vi "smartmeshIP serial mux IO.vi"(5 "tx_commandType":u8(ring) items=["subscribe"=22, "startNetwork"=45, "setUser"=58, "setTime"=54, "setNetworkConfig"=26, "setLicense"=56, "setIPConfig"=68, "setDownstreamFrameMode"=51, "setCommonJoinKey"=66, "setAdvertising"=50, "setACLEntry"=39, "sendIP"=59, "sendData"=44, "restorFactoryDefaults"=61, "reset"=21, "radiotestTx"=35, "radiotestRx"=37, "pingMote"=42, "getTime"=23, "getSystemInfo"=46, "radiotestStatistics"=38, "getPathInfo"=48, "getNextPath"=49, "getNextACLEntry"=40, "getNetworkInfo"=64, "getNetworkConfig"=63, "getMoteLinks"=70, "getMoteInfo"=62, "getMoteConfigByld"=65, "getMoteConfig"=47, "getManagerStatistics"=53, "getLog"=43, "getLicense"=55, "getIPConfig"=67, "exchangeNetworkID"=34, "exchangeMoteJoinKey"=33, "deleteMote"=69, "deleteACLEntry"=41, "clearStatistics"=31], 7 "State":u16(ring) items=["Connect", "Write", "Read", "Close"], 8 "error in":errorcluster, 9 "MAC source":string="\u0000\u0017\r\u0000\u0000`#Ò", 10 "tx_data":string, 11 "serial mux adress":T1={"serial_mux IP"="127.0.0.1", "rserial_mux port"=9900}) -> (0 "error out":errorcluster, 1 "tx packet":string, 2 "rx_commandType":u8, 3 "rx_data":string, 4 "all inputs":string[](array[string]), 6 "sec since last packet":dbl)   [LabVIEW 2017]
panel:
  in  "reset connection each month?":bool=TRUE
  out "Array 2":u8[](array[numeric])
  in  "MAC destination":string="\u0000\u0017\r\u0000\u0000`#Ò"
  in  "Path ID":u16
  in  "advertising":bool
  in  "next mote on list?":bool
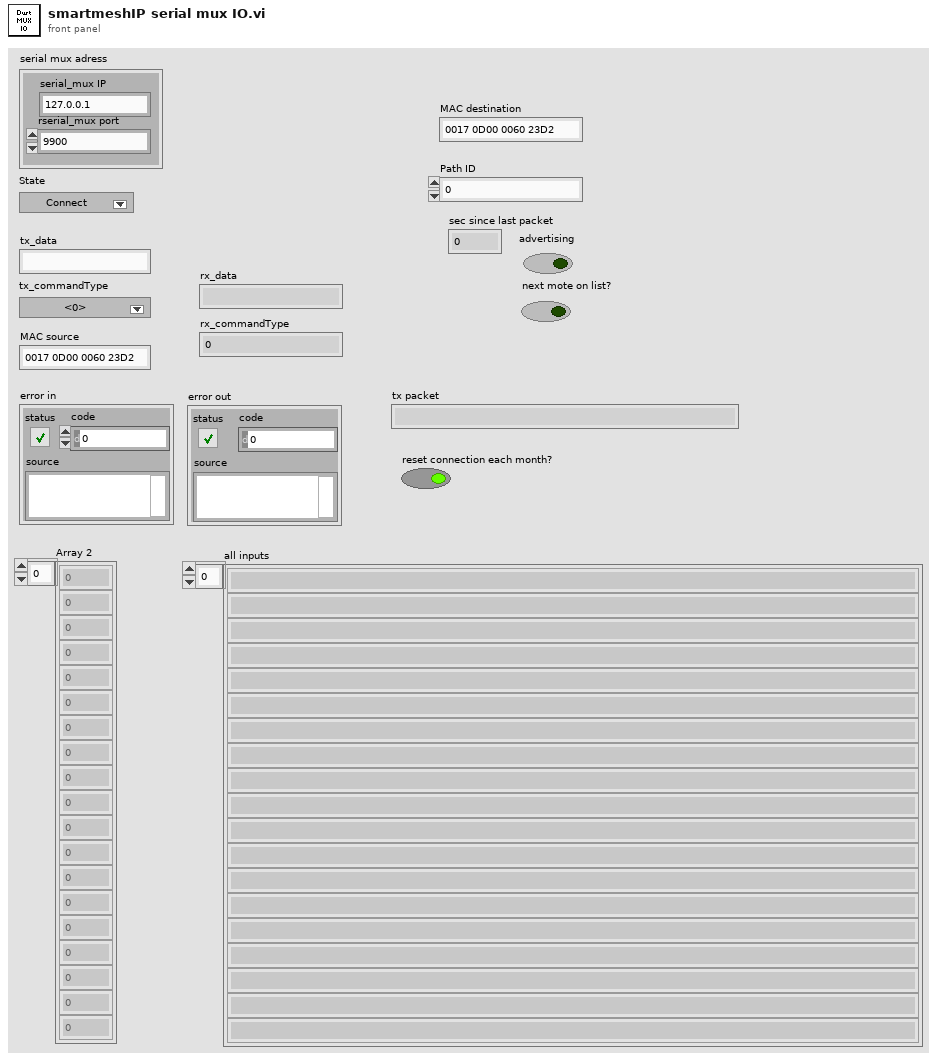
[diagram p1: front panel]
types:
  T1 = cluster{"serial_mux IP":string, "rserial_mux port":u16}
  T2 = enum16{"Standard", "Buffered", "CRLF", "Immediate"}
  T3 = typedef "LVDateTimeRec.ctl" = cluster{"fractional second":dbl, "second":i32, "minute":i32, "hour":i32, "day of month":i32, "month":i32, "year":i32, "day of week":i32, "day of year":i32, "DST":i32}
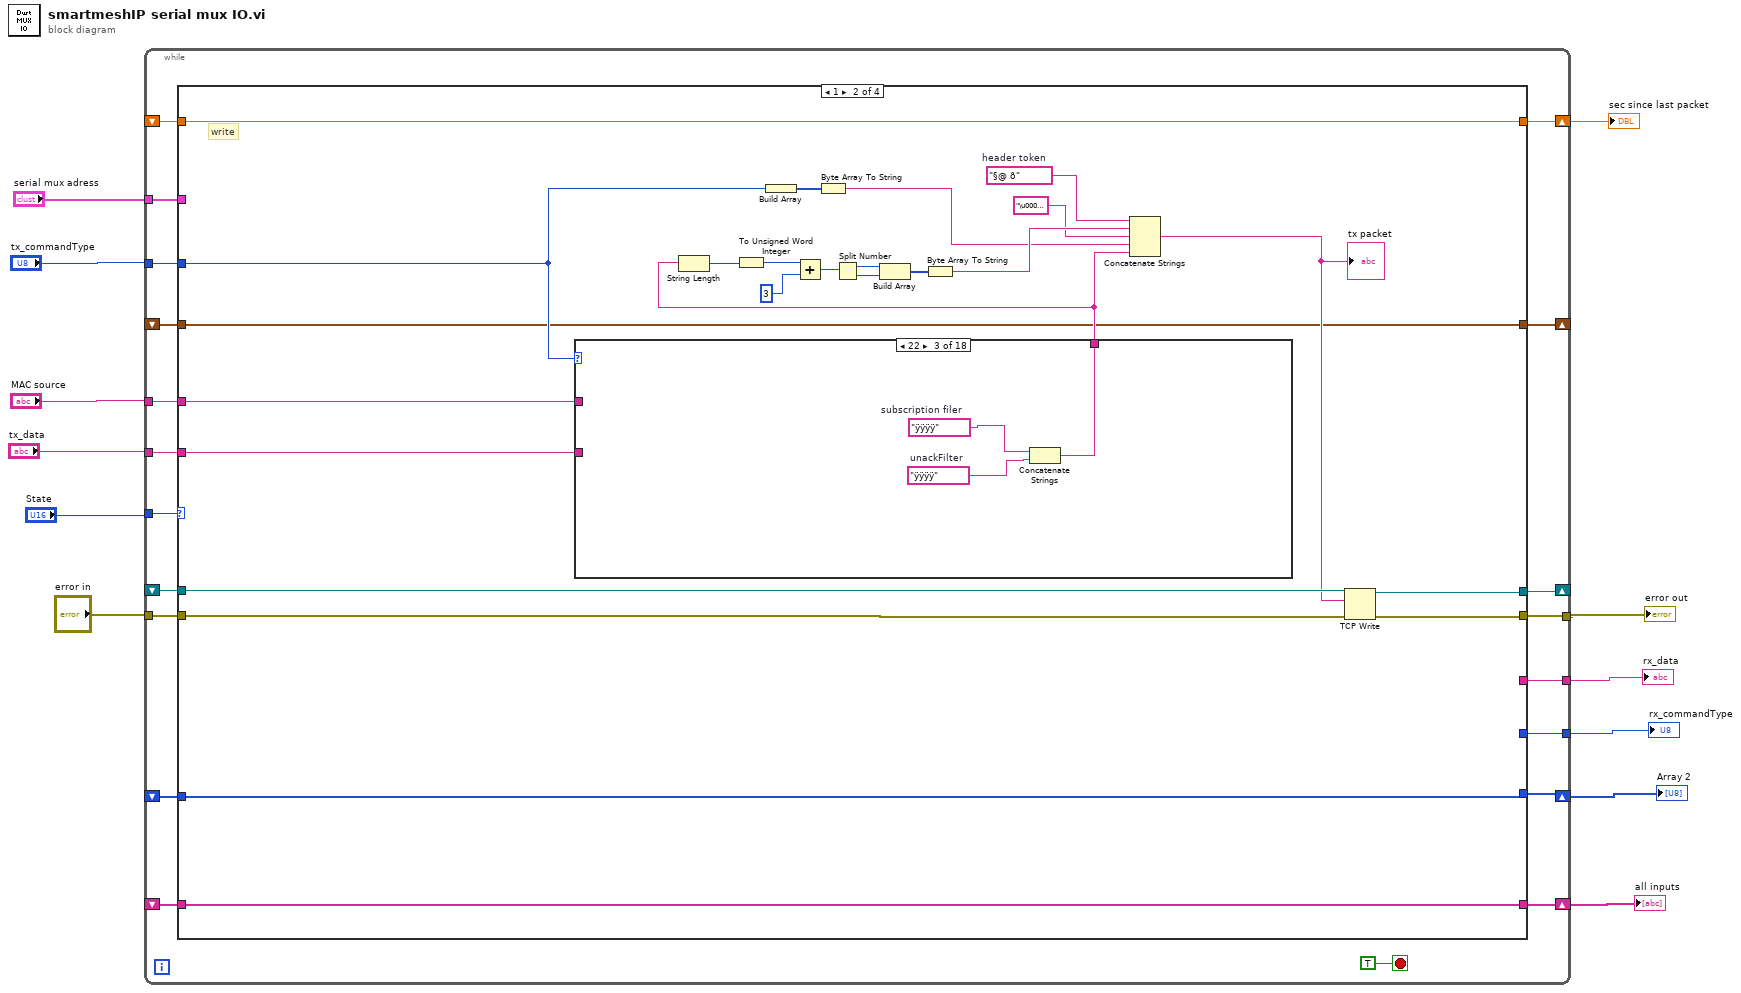
[diagram p0: block diagram]
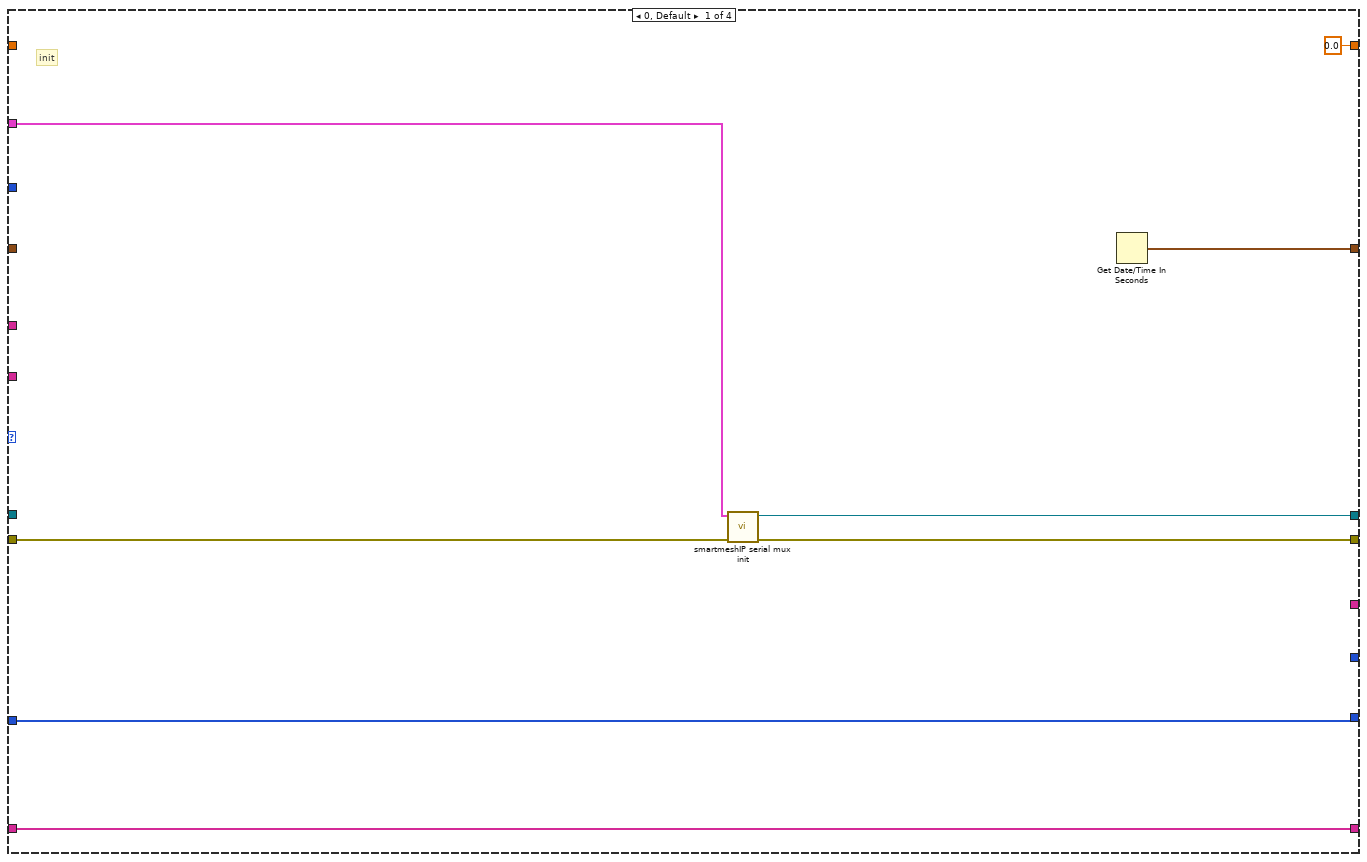
[diagram p2: hidden frame]
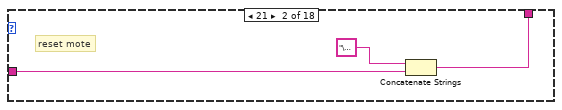
[diagram p4: hidden frame]
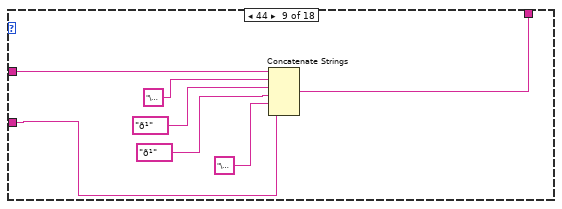
[diagram p10: hidden frame]
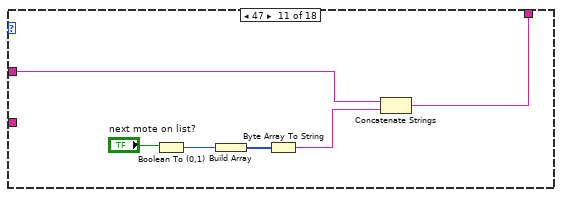
[diagram p12: hidden frame]
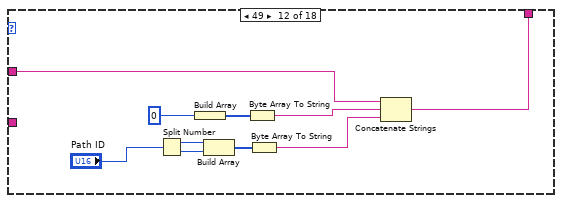
[diagram p13: hidden frame]
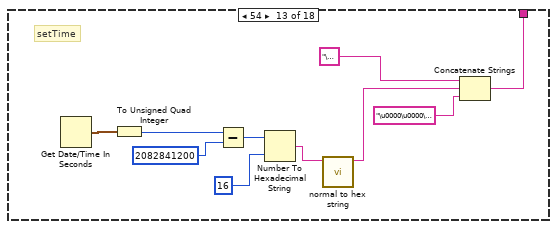
[diagram p14: hidden frame]
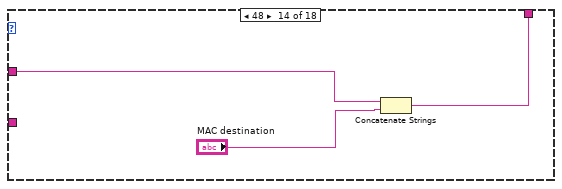
[diagram p15: hidden frame]
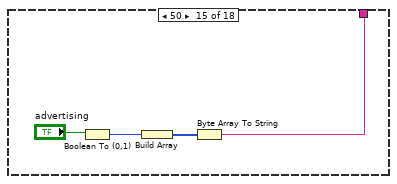
[diagram p16: hidden frame]
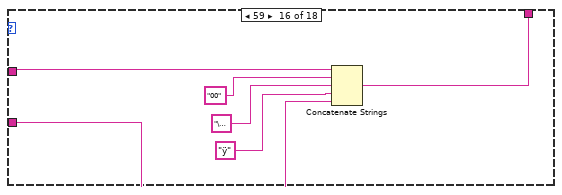
[diagram p17: hidden frame]
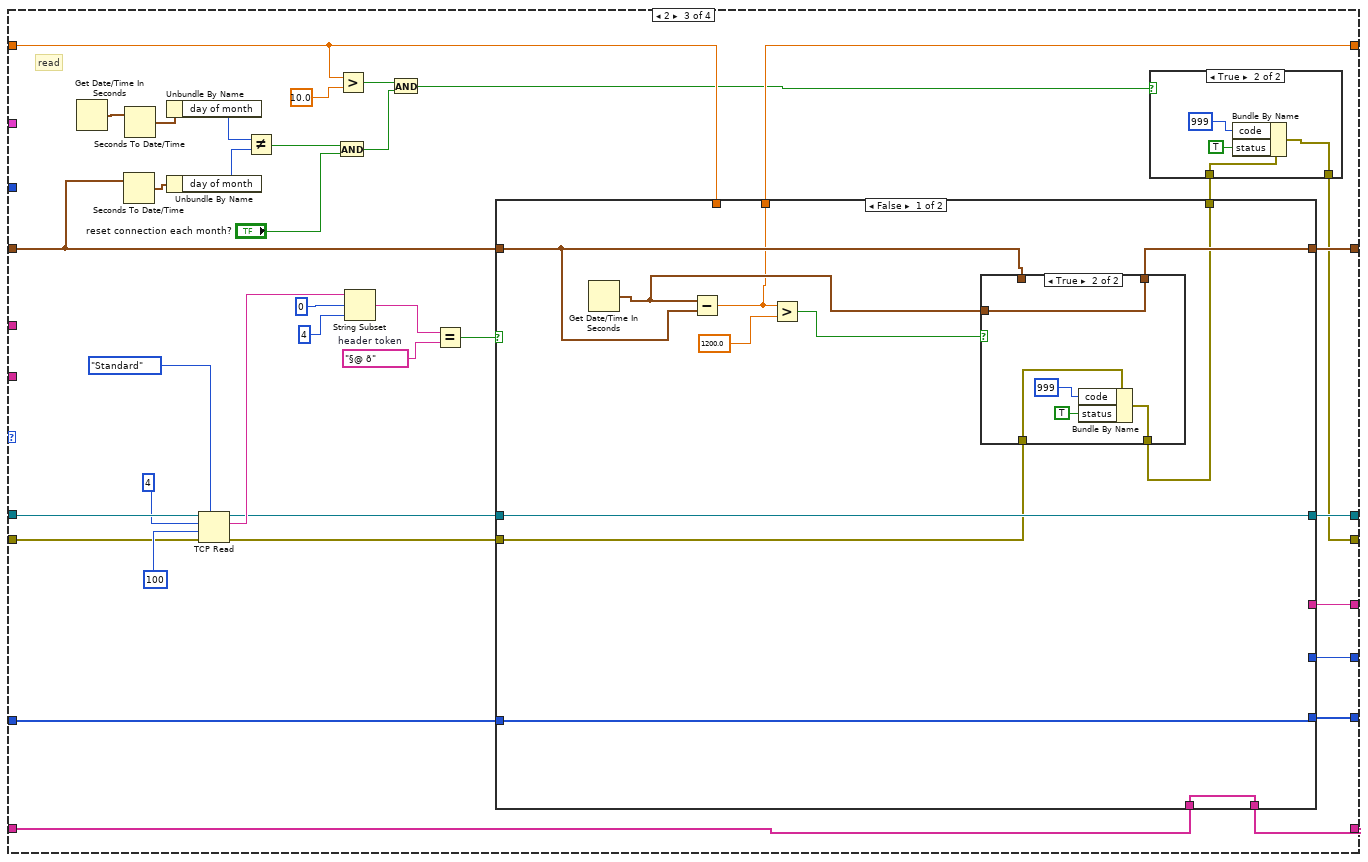
[diagram p20: hidden frame]
diagram:
  n1 = while {
    tunnel: "State" -> [w31]
    tunnel: [w30] -> w11
    shift-right: [w29] -> _
    shift-left: _ -> [w28]
    tunnel: "error in" -> [w27]
    tunnel: "tx_commandType" -> [w26]
    tunnel: [w25] -> w8
    tunnel: [w24] -> w7
    tunnel: "MAC source" -> [w23]
    tunnel: "tx_data" -> [w22]
    shift-right: [w21] -> w4
    shift-left: _ -> [w20]
    shift-right: [w19] -> w3
    shift-left: _ -> [w18]
    tunnel: "serial mux adress" -> [w17]
    shift-right: [w16] -> _
    shift-left: _ -> [w15]
    shift-right: [w14] -> w1
    shift-left: _ -> [w13]
    stop <- TRUE stop-if-true
    n2 = case shown="1" w31 {
      tunnel: [w37 w47 w125 w221] -> w30
      tunnel: [w36 w48 w143 _] -> w29
      tunnel: w28 -> [_ w64 w160 w222]
      tunnel: w27 -> [w38 w65 w145 w223]
      tunnel: w26 -> [_ w54 _ _]
      tunnel: [_ _ w152 _] -> w25
      tunnel: [_ _ w150 _] -> w24
      tunnel: w23 -> [_ w46 _ _]
      tunnel: w22 -> [_ w45 _ _]
      tunnel: [w40 w44 w148 w220] -> w21
      tunnel: w20 -> [w40 w44 w149 w220]
      tunnel: [w39 w43 w147 w219] -> w19
      tunnel: w18 -> [w39 w43 w146 w219]
      tunnel: w17 -> [w35 _ _ _]
      tunnel: [w34 w42 w142 w218] -> w16
      tunnel: w15 -> [_ w42 w136 w218]
      tunnel: [0.0 w41 w133 w217] -> w14
      tunnel: w13 -> [_ w41 w131 w217]
      frame 0, Default {
        # "init"
        n3 = call "smartmeshIP serial mux init.vi"("error in (no error)"=w38, "serial mux adress"=w35) -> ("error out"=w37:errorcluster, "connection ID out"=w36:refnum<k5>)  [unwired: 8 in]
        n4 = Get Date/Time In Seconds() -> (seconds since 1Jan1904=w34:timestamp)
      }
      frame 1 {
        w60 = "§@ õ"  # header token
        # "write"
        n5 = case shown="22" w54 {
          tunnel: w46 -> [_ w69 _ _ w73 w74 w75 w76 w83 _ w88 w99 _ w112 _ w119 w123 w124]
          tunnel: [w66 w68 w70 _ w73 w74 w75 w76 w81 _ w84 w96 w109 w111 w113 w118 w123 w124] -> w55
          tunnel: w45 -> [w66 _ _ _ _ _ _ _ w82 _ _ _ _ _ _ w117 _ _]
          frame 0, Default {
          }
          frame 21 {
            # "reset mote"
            n6 = Concatenate Strings("\u0002", w69) -> (w68:string)
          }
          frame 22 {
            w72 = "ÿÿÿÿ"  # unackFilter
            w71 = "ÿÿÿÿ"  # subscription filer
            n7 = Concatenate Strings(w71, w72) -> (w70:string)
          }
          frame 23 {
          }
          frame 40 {
          }
          frame 41 {
          }
          frame 42 {
          }
          frame 43 {
          }
          frame 44 {
            n8 = Concatenate Strings(w83, "\u0000" ("string"), "ð¹" ("string"), "ð¹" ("string"), "\u0000" ("string"), w82) -> (w81:string)
          }
          frame 45 {
          }
          frame 47 {
            n9 = Boolean To (0,1)(Boolean="next mote on list?") -> (0, 1=w87:i16)
            n10 = Build Array(w87) -> (w86:i16[])
            n11 = Byte Array To String(unsigned byte array=w86) -> (string=w85:string)
            n12 = Concatenate Strings(w88, w85) -> (w84:string)
          }
          frame 49 {
            n13 = Split Number(x="Path ID") -> (hi(x)=w94:u8, lo(x)=w93:u8)
            n14 = Build Array(u8 0 ("element")) -> (w98:u8[])
            n15 = Build Array(w94, w93) -> (w95:u8[])
            n16 = Byte Array To String(unsigned byte array=w98) -> (string=w97:string)
            n17 = Byte Array To String(unsigned byte array=w95) -> (string=w92:string)
            n18 = Concatenate Strings(w99, w97, w92) -> (w96:string)
          }
          frame 54 {
            # "setTime"
            n19 = Get Date/Time In Seconds() -> (seconds since 1Jan1904=w107:timestamp)
            n20 = To Unsigned Quad Integer(1:w107) -> (0:w105:u64)
            n21 = Subtract(x=w105, y=u64 2082841200 ("double precision float 2")) -> (x-y=w104:u64)
            n22 = Number To Hexadecimal String(1:i16 16 ("width (-)"), 2:w104) -> (0:w102:string)
            n23 = call "normal to hex string.vi"("Normal String"=w102) -> ("Hex Display Sting"=w101:string)  [unwired: 10 in]
            n24 = Concatenate Strings("\u0000" ("data in"), w101, "\u0000\u0000\u0000\u0000" ("data in")) -> (w109:string)
          }
          frame 48 {
            n25 = Concatenate Strings(w112, "MAC destination") -> (w111:string)
          }
          frame 50 {
            n26 = Boolean To (0,1)(Boolean="advertising") -> (0, 1=w115:i16)
            n27 = Build Array(w115) -> (w114:i16[])
            n28 = Byte Array To String(unsigned byte array=w114) -> (string=w113:string)
          }
          frame 59 {
            n29 = Concatenate Strings(w119, "00" ("string"), "\u0000" ("string"), "ÿ" ("string"), w117) -> (w118:string)
          }
          frame 62 {
          }
          frame 69 {
          }
        }
        n30 = String Length(string=w55) -> (length=w50:i32)
        n31 = To Unsigned Word Integer(number=w50) -> (unsigned 16bit integer=w49:u16)
        n32 = Build Array(w54) -> (w61:u8[])
        n33 = Add(x=w49, y=u16 3) -> (x+y=w53:u16)
        n34 = Byte Array To String(unsigned byte array=w61) -> (string=w57:string)
        n35 = Split Number(x=w53) -> (hi(x)=w52:u8, lo(x)=w51:u8)
        n36 = Build Array(w52, w51) -> (w62:u8[])
        n37 = Byte Array To String(unsigned byte array=w62) -> (string=w59:string)
        n38 = Concatenate Strings(w60, w59, "\u0000\u0000" ("data in"), w57, w55) -> (w56:string)
        "tx packet" <- w56
        n39 = TCP Write(connection ID=w64, data in=w56, error in (no error)=w65) -> (connection ID out=w48:refnum<k5>, error out=w47:errorcluster)  [unwired: 1 in, 1 out]
      }
      frame 2 {
        w155 = "§@ õ"  # header token
        # "read"
        n40 = Get Date/Time In Seconds() -> (seconds since 1Jan1904=w140:timestamp)
        n41 = Seconds To Date/Time(time stamp (now)=w136) -> (date time rec=w141:T3)  [unwired: 1 in]
        n42 = Seconds To Date/Time(time stamp (now)=w140) -> (date time rec=w137:T3)  [unwired: 1 in]
        n43 = Unbundle By Name(w137) -> ("day of month"=w138:i32)
        n44 = Unbundle By Name(w141) -> ("day of month"=w139:i32)
        n45 = TCP Read(connection ID=w160, bytes to read=4, error in (no error)=w145, 7:T2."Standard" ("mode (standard)"), 9:100 ("timeout ms (25000)")) -> (connection ID out=w144:refnum<k5>, data out=w156:string, error out=w127:errorcluster)
        n46 = Not Equal?(x=w138, y=w139) -> (x != y?=w135:bool)
        n47 = And(x=w135, y="reset connection each month?") -> (x .and. y?=w129:bool)
        n48 = Greater?(x=w131, y=10.0) -> (0:w130:bool)
        n49 = String Subset(string=w156, offset (0)=0, length (rest)=4 ("length (rest)")) -> (substring=w154:string)
        n50 = And(x=w130, y=w129) -> (x .and. y?=w128:bool)
        n51 = Equal?(x=w154, y=w155) -> (x = y?=w153:bool)
        n52 = case shown="False" w153 {
          tunnel: w127 -> [w172 w212]
          tunnel: [w173 w207] -> w143
          tunnel: w144 -> [w173 w211]
          tunnel: [_ w189] -> w152
          tunnel: [_ w194] -> w150
          tunnel: w149 -> [w177 w192]
          tunnel: [w177 w191] -> w148
          tunnel: [w176 w190] -> w147
          tunnel: w146 -> [w176 w188]
          tunnel: [w171 w187] -> w142
          tunnel: w136 -> [w169 _]
          tunnel: [w168 w186] -> w133
          tunnel: w131 -> [_ w186]
          tunnel: [w167 w185] -> w126
          frame False {
            n53 = Get Date/Time In Seconds() -> (seconds since 1Jan1904=w170:timestamp)
            n54 = Subtract(x=w170, y=w169) -> (x-y=w168:dbl)
            n55 = Greater?(x=w168, y=1200.0) -> (0:w174:bool)
            n56 = case shown="True" w174 {
              tunnel: w172 -> [w179 w184]
              tunnel: [w179 w183] -> w167
              tunnel: w169 -> [w178 _]
              tunnel: [w178 w181] -> w171
              tunnel: w170 -> [_ w181]
              frame False {
              }
              frame True {
                n57 = Bundle By Name(cluster=w184, "code"=999, "status"=TRUE) -> (w183:errorcluster)
              }
            }
          }
          frame True {
            n58 = TCP Read(connection ID=w211, bytes to read=5, error in (no error)=w212) -> (connection ID out=w208:refnum<k5>, data out=w193:string, error out=w209:errorcluster)  [unwired: 2 in]
            n59 = String Subset(string=w193, offset (0)=0, length (rest)=2 ("length (rest)")) -> (substring=w204:string)
            n60 = String Subset(string=w193, offset (0)=4, length (rest)=1 ("length (rest)")) -> (substring=w197:string)
            n61 = String To Byte Array(string=w197) -> (unsigned byte array=w196:u8[])
            n62 = String To Byte Array(string=w204) -> (unsigned byte array=w202:u8[])
            n63 = Index Array(array=w196, index=0) -> (element=w189:u8)
            n64 = Index Array(array=w202, index=1) -> (element=w200:u8)
            n65 = Index Array(array=w202, index=0) -> (element=w199:u8)
            n66 = Join Numbers(hi=w199, lo=w200) -> ((hi.lo)=w198:u16)
            n67 = Subtract(x=w198, y=u16 3) -> (x-y=w205:u16)
            n68 = TCP Read(connection ID=w208, bytes to read=w205, error in (no error)=w209) -> (connection ID out=w207:refnum<k5>, data out=w194:string, error out=w185:errorcluster)  [unwired: 2 in]
            n69 = Build Array (concatenate)(w194, w192) -> (w191:string[])
            n70 = Get Date/Time In Seconds() -> (seconds since 1Jan1904=w187:timestamp)
            n71 = Build Array (concatenate)(w189, w188) -> (w190:u8[])
          }
        }
        n72 = case shown="True" w128 {
          tunnel: w126 -> [w162 w163]
          tunnel: [w162 w164] -> w125
          frame False {
          }
          frame True {
            n73 = Bundle By Name(cluster=w163, "code"=999, "status"=TRUE) -> (w164:errorcluster)
          }
        }
      }
      frame 3 {
        # "close"
        n74 = TCP Close Connection(connection ID=w222, error in (no error)=w223) -> (error out=w221:errorcluster)  [unwired: 1 in, 1 out]
      }
    }
  }
  "error out" <- w11
  "rx_commandType" <- w8
  "rx_data" <- w7
  "all inputs" <- w4
  "Array 2" <- w3
  "sec since last packet" <- w1
